vi "_STA_.vi"(0 "System no.":i32=1 min=1 max=4 step=1, 2 "Axes to query":string[](array[string]), 3 "All axes?":bool, 4 "Axis identifier?":bool=TRUE, 5 "error in":errorcluster) -> (14 "Axis status":dbl[](array[numeric]), 19 "error out":errorcluster)   [LabVIEW 2014]
doc: "Returns axis status (integer). Required by \"General wait for movement to stop.vi\" and \"Wait for axes to stop.vi\".\n\nValid for C-702, C-848, C-880, C-880K005, M-8X0 (but must be present in Special command.llb for all other systems, too)\n\nC702: If All axes = TRUE, then Axis identifier can be FALSE\nC-848: If All axes = TRUE, then Axis identifier can be FALSE\nC-880: If All axes = TRUE, then Axis identifier can be FALSE\nC-880K005: VI only supported when called through PI_Multix.vi\nM-8X0: M-8X0: All axes? = TRUE, Axis identifier? = FALSE. Check HELP answer to find out if STA? is supported. Command is equivalent to #4."
panel:
  # "Returns axis status (integer)."
  # "If all axes: use"
  # "Query"
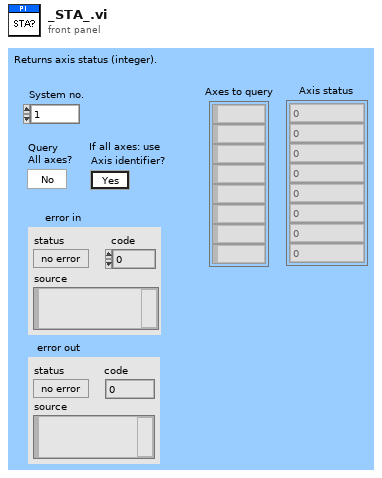
[diagram p1: front panel]
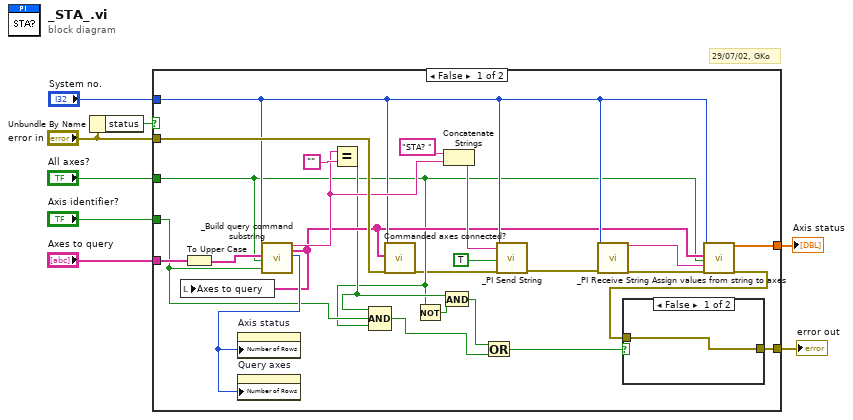
[diagram p0: block diagram]
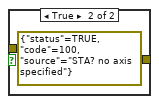
[diagram p2: hidden frame]
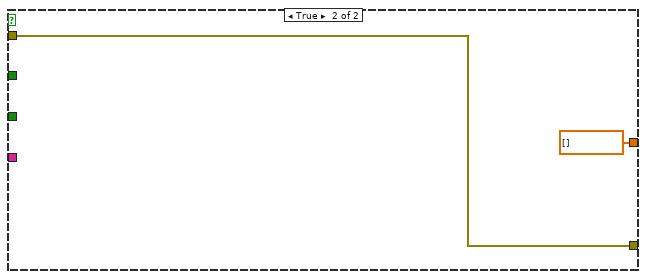
[diagram p3: hidden frame]
diagram:
  # "29/07/02, GKo"
  n1 = Unbundle By Name("error in") -> ("status"=w2:bool)
  n2 = case shown="False" w2 {
    tunnel: [w29 dbl[] [] ("Values")] -> w8
    tunnel: "error in" -> [w28 w37]
    tunnel: "Axes to query" -> [w27 _]
    tunnel: [w25 w37] -> w6
    tunnel: "System no." -> [w21 _]
    tunnel: "Axis identifier?" -> [w13 _]
    tunnel: "All axes?" -> [w12 _]
    frame False {
      n3 = To Upper Case(1:w27) -> (0:w24:string[])
      n4 = call "_Build query command substring.vi"("System no."=w21, "Axes to query in"=w24, "Query\nAll axes?"=w12, "For all axes: use\nAxis identifier?"=w13) -> ("Command substring"=w23:string, "Axes to query out"=w20:string[], "Number of rows"=w22:u32)  [unwired: 13 in]
      n5 = local write "Axes to query"(w20) -> ()
      n6 = property on="Axis status" class="Arr (strict)"("Number of Rows"=w22) -> ()  [unwired: 2 in, 2 out]
      n7 = property on="Query axes" class="Arr (strict)"("Number of Rows"=w22) -> ()  [unwired: 2 in, 2 out]
      n8 = Equal?(x=w23, y="" ("x")) -> (x = y?=w14:bool)
      n9 = Compound Arithmetic op=AND(w14, w13, w12) -> (w11:bool)
      n10 = call "Commanded axes connected?.vi"("System no."=w21, "Commanded axes"=w20, "error in"=w28) -> ("error out"=w10:errorcluster)  [unwired: 15 in, 1 out]
      n11 = Not(x=w12) -> (.not. x?=w17:bool)
      n12 = And(x=w14, y=w17) -> (x .and. y?=w15:bool)
      n13 = Concatenate Strings("STA? ", w23) -> (w30:string)
      n14 = Or(x=w15, y=w11) -> (x .or. y?=w16:bool)
      n15 = call "_PI Send String.vi"("System no."=w21, "String to send"=w30, "Attach termination char.?"=TRUE ("Attach Linefeed?"), "error in"=w10) -> ("error out"=w33:errorcluster)  [unwired: 15 in]
      n16 = call "_PI Receive String.vi"("System no."=w21, "error in"=w33) -> ("String read"=w19:string, "error out"=w9:errorcluster)  [unwired: 15 in, 1 out]
      n17 = call "Assign values from string to axes.vi"("System no."=w21, "Queried axes"=w20, "All axes queried?"=w12, "Input String"=w19, "error in"=w9) -> ("Values"=w29:dbl[], "error out"=w18:errorcluster)  [unwired: 11 in, 2 out]
      n18 = case shown="False" w16 {
        tunnel: [w34 errorcluster {"status"=TRUE, "code"=100, "source"="STA? no axis specified"} ("error out")] -> w25
        tunnel: w18 -> [w34 _]
        frame False {
        }
        frame True {
        }
      }
    }
    frame True {
    }
  }
  "error out" <- w6
  "Axis status" <- w8
